vi "AAL Resample (Const to Variable).vi"(7 "reset? (True)":bool=TRUE, 8 "error in (no error)":errorcluster, 9 "config":T1={"timing jitter"=enum."Interpolation", "anti-aliasing?"=TRUE, "filter prototype"={"coefficients"=[], "factor"=1}} {"filter prototype"."coefficients" format="%.2f"}, 10 "time":dbl[](array[numeric]) format="%.2f", 11 "X":dbl[](array[numeric])) -> (0 "error out":errorcluster, 1 "offset":i32, 2 "time stamps":dbl[](array[numeric]) format="%.2f", 3 "Y":dbl[](array[numeric]) format="%.2f")   [LabVIEW 2010, in "NI_AALPro.lvlib"]
doc: "Perform an arbitrary resampling on the input signal."
uses:
  NI_AALPro.lvlib
  lvanlys.dll
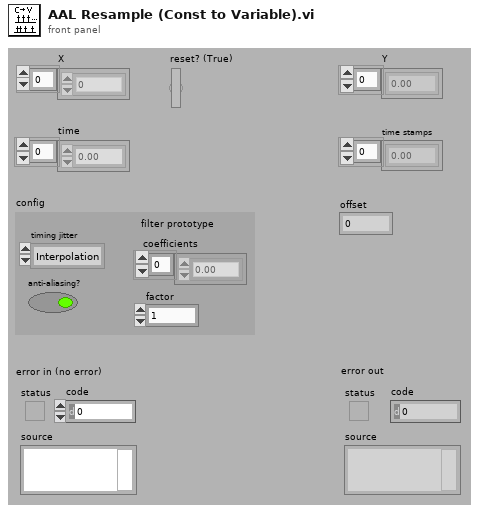
[diagram p1: front panel]
types:
  T1 = cluster{"timing jitter":enum32{"Interpolation", "Rounding"}, "anti-aliasing?":bool, "filter prototype":cluster{"coefficients":dbl[], "factor":i32}}
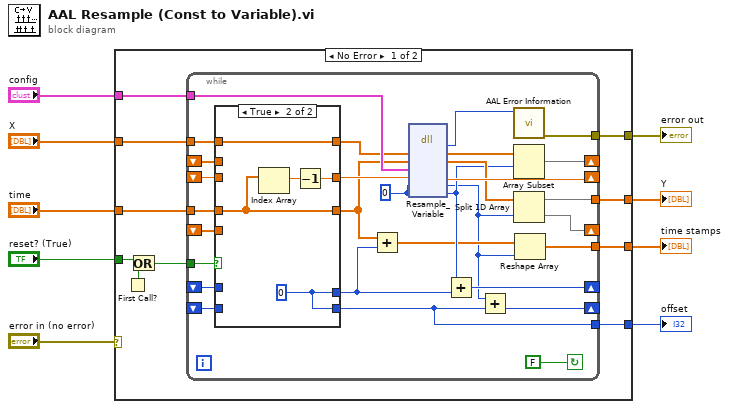
[diagram p0: block diagram]
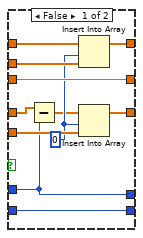
[diagram p2: hidden frame]
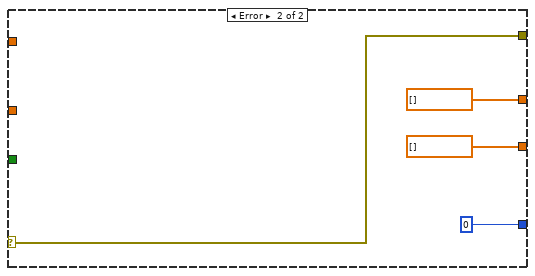
[diagram p3: hidden frame]
diagram:
  n1 = case shown="No Error" "error in (no error)" {
    selector: "error in (no error)" -> [_ w69]
    tunnel: "config" -> [w18 _]
    tunnel: "reset? (True)" -> [w17 _]
    tunnel: "time" -> [w11 _]
    tunnel: [w15 dbl[] []] -> w6
    tunnel: [w14 dbl[] []] -> w5
    tunnel: [w13 0] -> w4
    tunnel: [w12 w69] -> w3
    tunnel: "X" -> [w10 _]
    frame No Error {
      n2 = First Call?() -> (First Call?: T/F=w19:bool)
      n3 = Or(x=w17, y=w19) -> (x .or. y?=w16:bool)
      n4 = while {
        tunnel: [w34] -> w14
        tunnel: [w20] -> w15
        shift-right: [w47] -> _
        shift-left: _ -> [w39]
        shift-right: [w48] -> _
        shift-left: _ -> [w40]
        tunnel: w10 -> [w44]
        tunnel: w11 -> [w42]
        shift-right: [w46] -> _
        shift-left: _ -> [w38]
        tunnel: w16 -> [w37]
        tunnel: w18 -> [w49]
        shift-right: [w32] -> _
        shift-left: _ -> [w35]
        tunnel: [w24] -> w13
        shift-right: [w23] -> _
        shift-left: _ -> [w27]
        tunnel: [w21] -> w12
        stop <- FALSE continue-if-true
        w29 = 0
        n5 = case shown="True" w37 {
          tunnel: [w59 w65] -> w43
          tunnel: w44 -> [w57 w65]
          tunnel: [w54 w64] -> w31
          tunnel: w42 -> [w53 w64]
          tunnel: [w60 w62] -> w41
          tunnel: w40 -> [w56 _]
          tunnel: w39 -> [w58 _]
          tunnel: w38 -> [w60 _]
          tunnel: w35 -> [w51 _]
          tunnel: [w51 w61] -> w25
          tunnel: w27 -> [w50 _]
          tunnel: [w50 w61] -> w24
          frame False {
            w55 = 0 ("Index")
            n6 = Subtract(x=w53, y=w51) -> (x-y=w52:dbl[])
            n7 = Insert Into Array(array=w57, index=w55, new element=w56) -> (w59:dbl[])
            n8 = Insert Into Array(array=w52, index=w55, new element=w58) -> (w54:dbl[])
          }
          frame True {
            w61 = 0
            n9 = Index Array(array=w64) -> (element=w63:dbl)  [unwired: 1 in]
            n10 = Decrement(x=w63) -> (x-1=w62:dbl)
          }
        }
        n11 = Add(x=w31, y=w25) -> (x+y=w30:dbl[])
        n12 = dll-call lib="C:/Program Files/National Instruments/LabVIEW 2010/resource/lvanlys.*" fn="Resample_Variable"("xH"=w43, "timeH"=w31, "config"=w49, "last_sample_time"=w41, "out_len"=w29, "xLeftOverIdx"=w29) -> (w22:i32, "xH"=w28:dbl[], "timeH"=w36:dbl[], "last_sample_time"=w46:dbl, "out_len"=w26:i32, "xLeftOverIdx"=w33:i32)  [unwired: 4 in, 2 out]
        n13 = Add(x=w33, y=w25) -> (x+y=w32:i32)
        n14 = Add(x=w26, y=w24) -> (x+y=w23:i32)
        n15 = call "AAL Error Information.vi"("error code"=w22) -> ("error out"=w21:errorcluster)  [unwired: 10 in]
        n16 = Array Subset(array=w28, index=w33) -> (w48:dbl[])  [unwired: 1 in]
        n17 = Split 1D Array(array=w36, index=w26) -> (first subarray=w34:dbl[], second subarray=w47:dbl[])
        n18 = Reshape Array(w30, w26) -> (w20:dbl[])
      }
    }
    frame Error {
    }
  }
  "time stamps" <- w6
  "Y" <- w5
  "offset" <- w4
  "error out" <- w3
